vi "ModbusErrorHandler.vi"(9 "connection error":bool, 11 "device in":T1) -> (3 "device out":T1)   [LabVIEW 2017, in "ModbusMaster.lvlib"]
uses:
  <vilib>/addons/InsightCM/Devices/Shared/Common/ModbusMaster/ModbusMaster.lvlib
  <vilib>/addons/InsightCM/Devices/Shared/Common/ModbusMaster/controls/ModbusDevice.ctl
  <vilib>/Modbus/master/Modbus Master.lvclass
  <vilib>/addons/InsightCM/Devices/Shared/Common/ModbusMaster/controls/ModbusChannel.ctl
  <vilib>/addons/InsightCM/Devices/Shared/Common/ModbusMaster/controls/RegisterType.ctl
  <vilib>/addons/InsightCM/MessageBus/Base/controls/DataSource.ctl
  <vilib>/addons/InsightCM/MessageBus/Base/controls/KeyValuePair.ctl
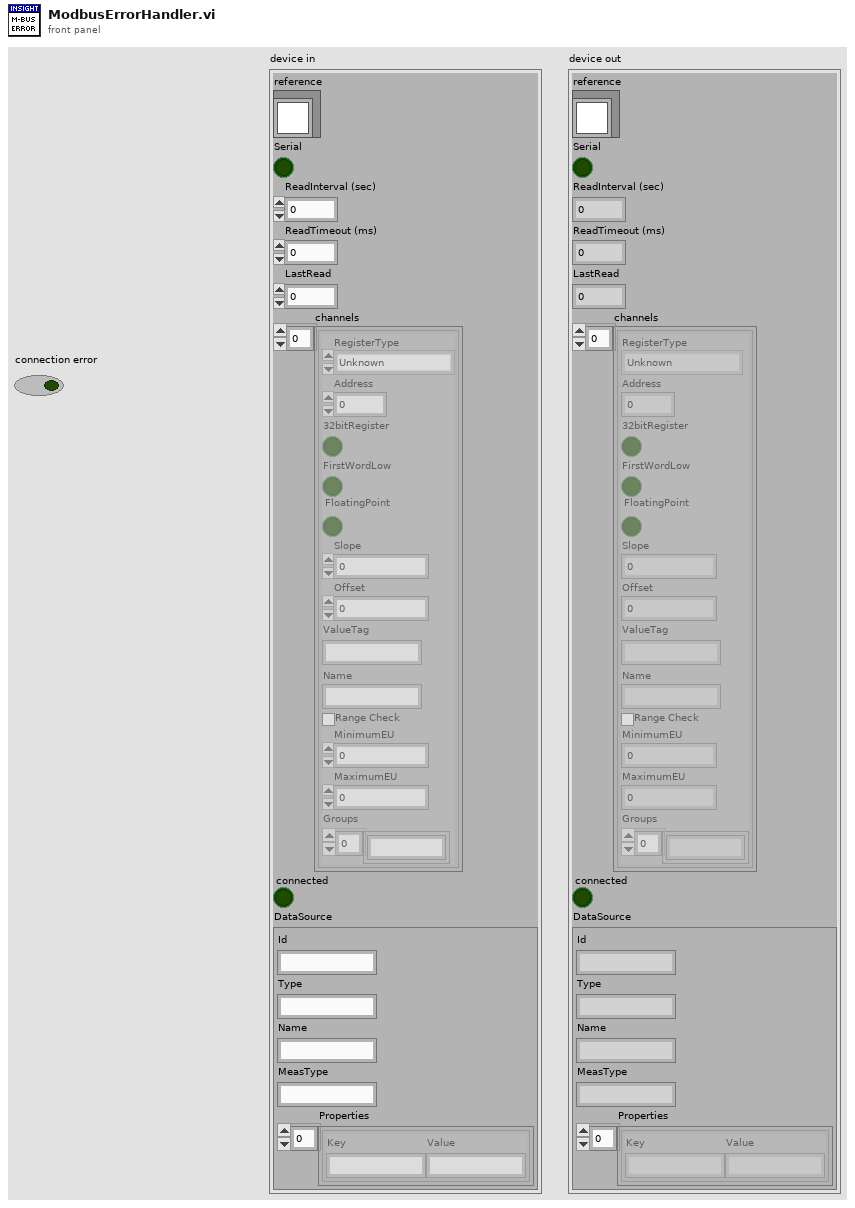
[diagram p1: front panel]
types:
  T1 = typedef "ModbusMaster.lvlib/ModbusDevice.ctl" = cluster{"reference":refnum<class "Modbus Master.lvclass">, "Serial":bool, "ReadInterval (sec)":dbl, "ReadTimeout (ms)":i32, "LastRead":dbl, "channels":T2[], "connected":bool, "DataSource":T4}
  T2 = typedef "ModbusMaster.lvlib/ModbusChannel.ctl" = cluster{"RegisterType":T3, "Address":i32, "32bitRegister":bool, "FirstWordLow":bool, "FloatingPoint":bool, "Slope":dbl, "Offset":dbl, "ValueTag":string, "Name":string, "Range Check":bool, "MinimumEU":dbl, "MaximumEU":dbl, "Groups":string[]}
  T3 = typedef "ModbusMaster.lvlib/RegisterType.ctl" = enum16{"Unknown", "Coil", "Discrete Input", "Holding Register", "Input Register"}
  T4 = typedef "DataSource.ctl" = cluster{"Id":string, "Type":string, "Name":string, "MeasType":string, "Properties":T5[]}
  T5 = typedef "KeyValuePair.ctl" = cluster{"Key":string, "Value":string}
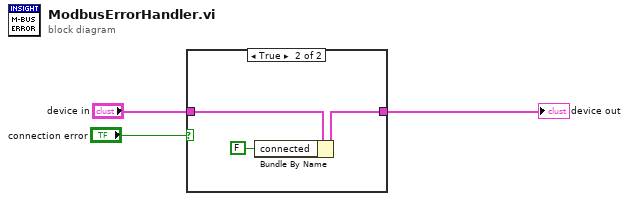
[diagram p0: block diagram]
diagram:
  n1 = case shown="True" "connection error" {
    tunnel: "device in" -> [w4 w7]
    tunnel: [w4 w6] -> w3
    frame False {
    }
    frame True {
      n2 = Bundle By Name(cluster=w7, "connected"=FALSE) -> (w6:T1)
    }
  }
  "device out" <- w3
